vi "DecodeString.vi"(1 "Array":bool[](array[boolean])) -> (0 "string 2":string)   [LabVIEW 2016]
uses:
  <vilib>/Utility/error.llb/whitespace.ctl
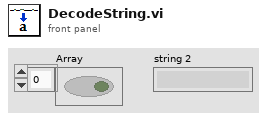
[diagram p1: front panel]
types:
  T1 = typedef "whitespace.ctl" = u16
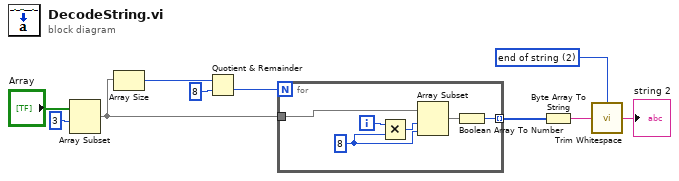
[diagram p0: block diagram]
diagram:
  w9 = T1 2 items=["both", "start of string", "end of string"] ("location (both)")
  n1 = Array Subset(array="Array", index=3) -> (w6:bool[])  [unwired: 1 in]
  n2 = Array Size(array=w6) -> (size(s)=w1:i32)
  n3 = Quotient & Remainder(x=w1, y=8) -> (floor(x/y)=w4:i32)  [unwired: 1 out]
  n4 = for {
    N: w4 -> [_]
    tunnel: w6 -> [w15]
    tunnel: [w12] -> w3 mode=indexing
    i -> [w11]
    w14 = 8 ("y")
    n5 = Multiply(x=w11, y=w14) -> (x*y=w16:i32)
    n6 = Array Subset(array=w15, index=w16, length=w14) -> (w13:bool[])
    n7 = Boolean Array To Number(Boolean array=w13) -> (number=w12:u8)
  }
  n8 = Byte Array To String(unsigned byte array=w3) -> (string=w8:string)
  n9 = call <vilib>:"Trim Whitespace.vi"("string"=w8, "location (both)"=w9) -> ("trimmed string"=→"string 2":string)
